vi "CtrlTreeCheckSelection.vi"(8 "error in (no error)":errorcluster, 11 "TreeControl in":refnum<vi>) -> (0 "error out":errorcluster, 3 "TreeControl out":refnum<vi>)   [LabVIEW 2020]
uses:
  5ef8c3ed-0c3b-457e-93ce-58833155010e.vi
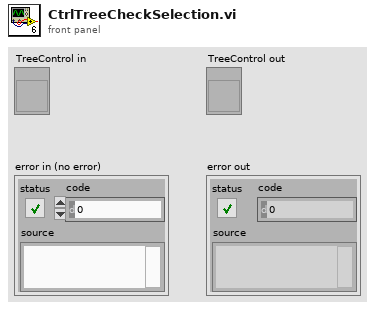
[diagram p1: front panel]
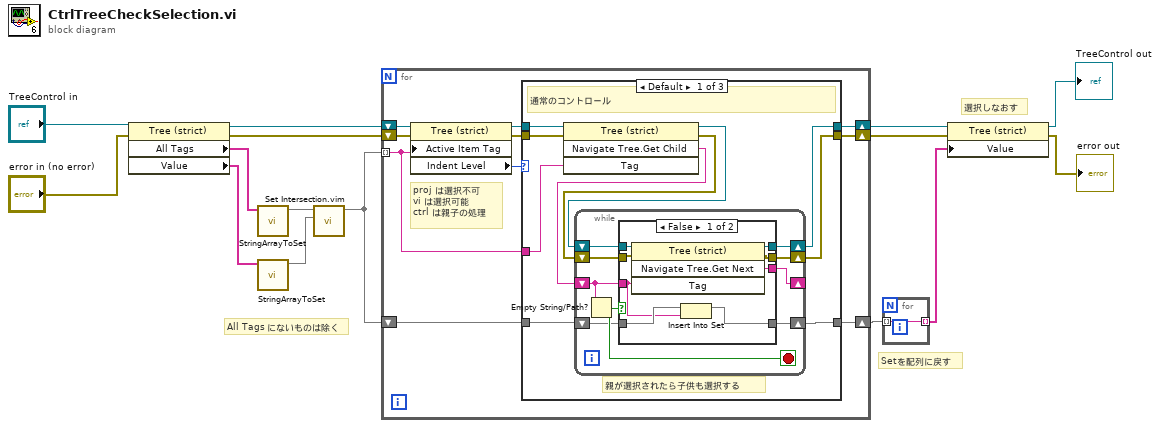
[diagram p0: block diagram]
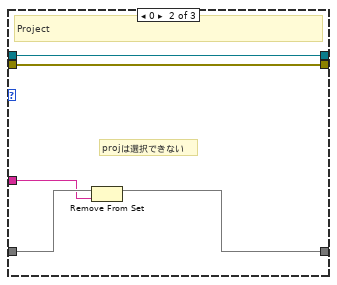
[diagram p3: hidden frame]
diagram:
  # "選択しなおす"
  # "Setを配列に戻す"
  # "All Tags にないものは除く"
  n1 = property class="Tree (strict)"(reference="TreeControl in", error in="error in (no error)") -> (reference out=w10:refnum<vi>, error out=w4:errorcluster, "All Tags"=w14:string[], "Value"=w7:string[])
  n2 = call "StringArrayToSet.vi"("String Array"=w14) -> ("Set"=w9:set{string})  [unwired: 10 in]
  n3 = call "StringArrayToSet.vi"("String Array"=w7) -> ("Set"=w8:set{string})  [unwired: 10 in]
  n4 = call "Set Intersection.vim"("set 2"=w8, "set 1"=w9) -> ("intersection"=w11:set{string})  [unwired: 9 in]
  n5 = for {
    shift-right: [w22] -> w13
    shift-left: w11 -> [w24]
    tunnel: w11 -> [w23] mode=indexing
    shift-right: [w20] -> w12
    shift-left: w10 -> [w25]
    shift-right: [w17] -> w3
    shift-left: w4 -> [w19]
    # "proj は選択不可\nvi は選択可能\nctrl は親子の処理"
    n6 = property class="Tree (strict)"(reference=w25, error in=w19, "Active Item Tag"=w23) -> (reference out=w21:refnum<vi>, error out=w18:errorcluster, "Indent Level"=w16:i32)
    n7 = case shown="Default" w16 {
      tunnel: w24 -> [w31 w61 w64]
      tunnel: w23 -> [w34 w60 _]
      tunnel: [w30 w59 w64] -> w22
      tunnel: w21 -> [w35 w58 w63]
      tunnel: [w29 w58 w63] -> w20
      tunnel: w18 -> [w28 w57 w62]
      tunnel: [w26 w57 w62] -> w17
      frame Default {
        # "親が選択されたら子供も選択する"
        # "通常のコントロール"
        n8 = invoke class="Tree (strict)" method="Navigate Tree.Get Child"(reference=w35, error in=w28, "Tag"=w34) -> (reference out=w32:refnum<vi>, error out=w27:errorcluster, "Navigate Tree:Get Child"=w33:string)  [unwired: 1 in, 1 out]
        n9 = while {
          shift-right: [w41] -> _
          shift-left: w33 -> [w44]
          shift-right: [w42] -> w29
          shift-left: w32 -> [w43]
          shift-right: [w38] -> w30
          shift-left: w31 -> [w39]
          shift-right: [w36] -> w26
          shift-left: w27 -> [w37]
          stop <- w40 stop-if-true
          n10 = Empty String/Path?(string/path=w44) -> (empty?=w40:bool)
          n11 = case shown="False" w40 {
            tunnel: w44 -> [w48 w55]
            tunnel: w43 -> [w52 w56]
            tunnel: [w51 w56] -> w42
            tunnel: [w50 w55] -> w41
            tunnel: w39 -> [w49 w54]
            tunnel: [w47 w54] -> w38
            tunnel: w37 -> [w46 w53]
            tunnel: [w45 w53] -> w36
            frame False {
              n12 = invoke class="Tree (strict)" method="Navigate Tree.Get Next"(reference=w52, error in=w46, "Tag"=w48) -> (reference out=w51:refnum<vi>, error out=w45:errorcluster, "Navigate Tree:Get Next Item"=w50:string)  [unwired: 1 in, 1 out]
              n13 = Insert Into Set(10:w48, 11:w49) -> (3:w47:set{string})  [unwired: 1 out]
            }
            frame True {
            }
          }
        }
      }
      frame 0 {
        # "projは選択できない"
        # "Project"
        n14 = Remove From Set(10:w60, 11:w61) -> (3:w59:set{string})  [unwired: 1 out]
      }
      frame 1 {
        # "vi は選択可能"
        # "VI"
      }
    }
  }
  n15 = for {
    tunnel: [w65] -> w15 mode=indexing
    tunnel: w13 -> [w65] mode=indexing
  }
  n16 = property class="Tree (strict)"(reference=w12, error in=w3, "Value"=w15) -> (reference out=→"TreeControl out":refnum<vi>, error out=→"error out":errorcluster)
